vi "NT to Globals & XML.vi"(8 "Array":path[](array[path])) -> ()   [LabVIEW 2020]
uses:
  NT to XML Number.vi
  Globals/Dashboard_Cal_Globals.vi
  2021-MARS-Swerve/Globals/Intake_Globals.vi
panel:
  in  "NT Name Categories":string[](array[string])=["Turret", "Intake", "Magazine", "Flywheel", "FR", "FL", "BL", "BR", "Manual", "Cowl"]
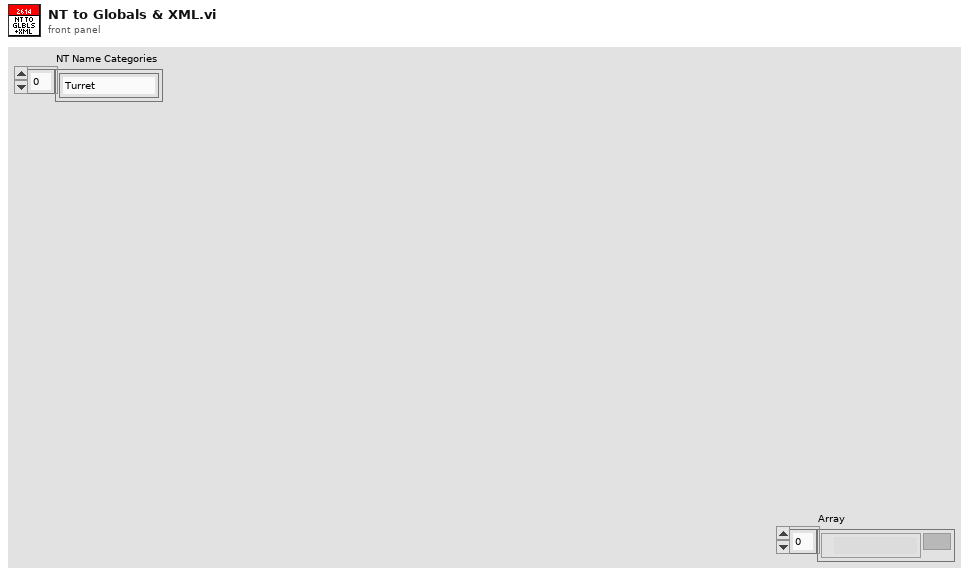
[diagram p1: front panel]
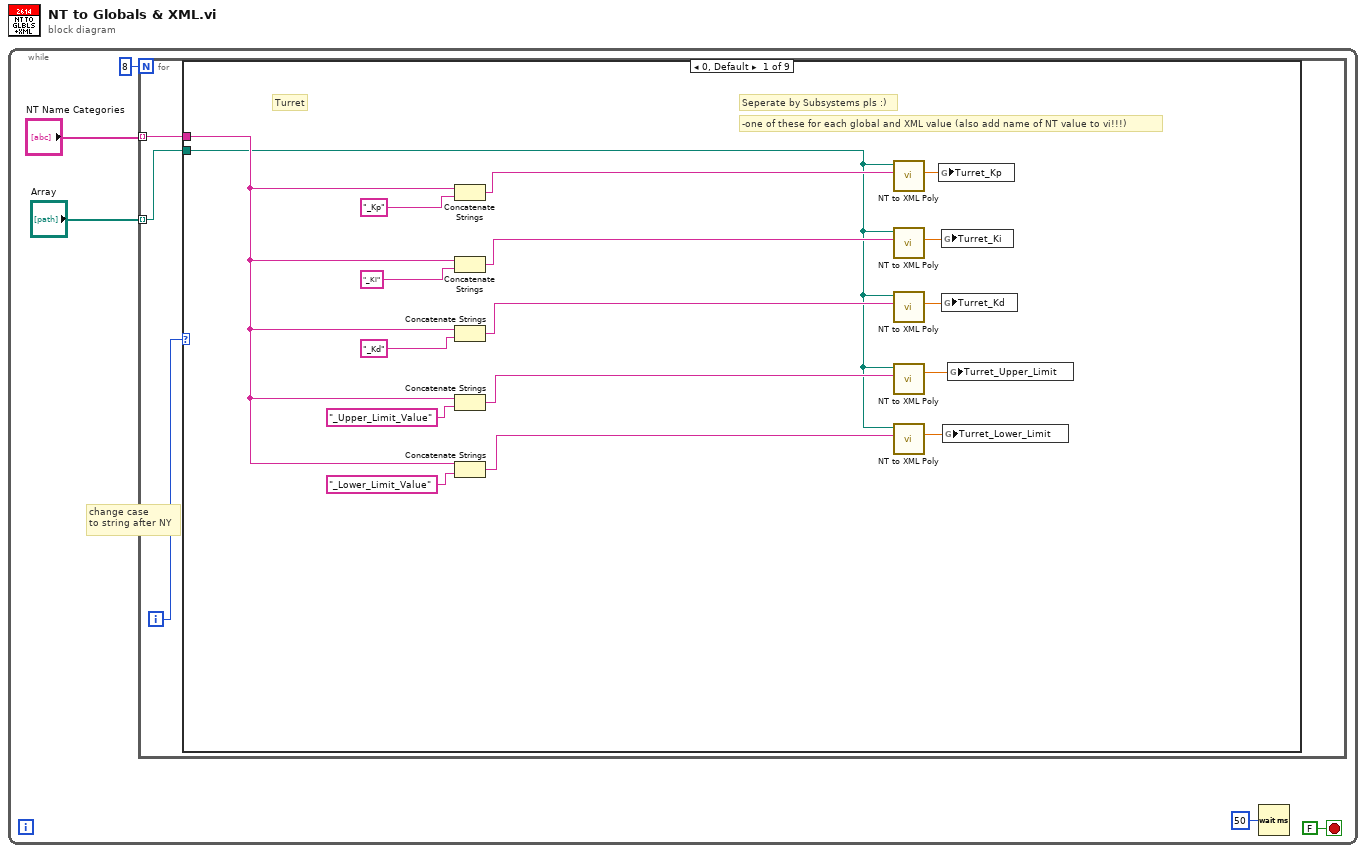
[diagram p0: block diagram]
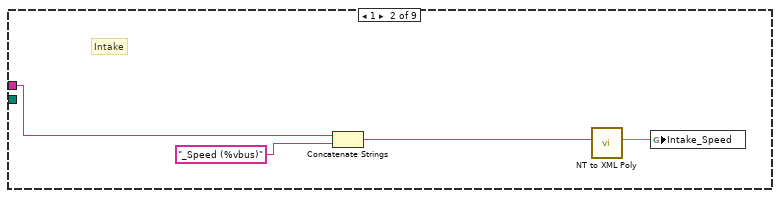
[diagram p2: hidden frame]
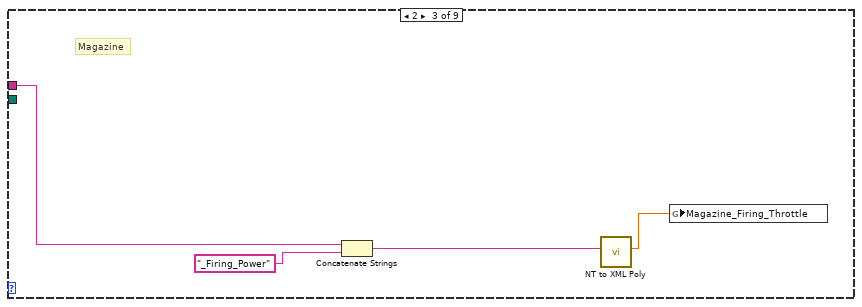
[diagram p3: hidden frame]
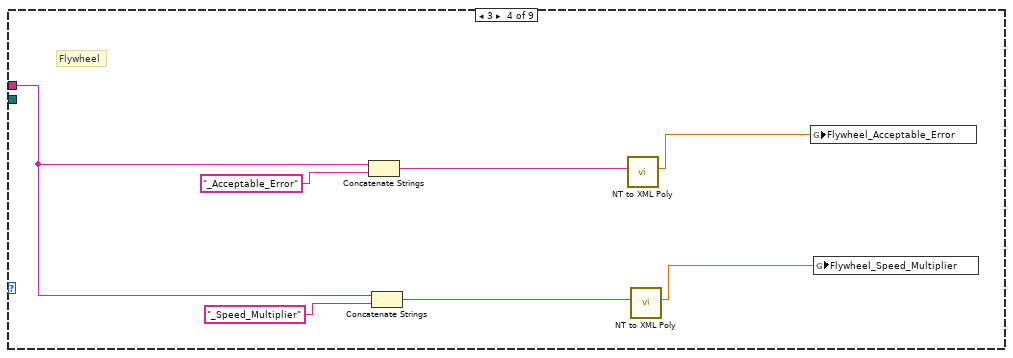
[diagram p4: hidden frame]
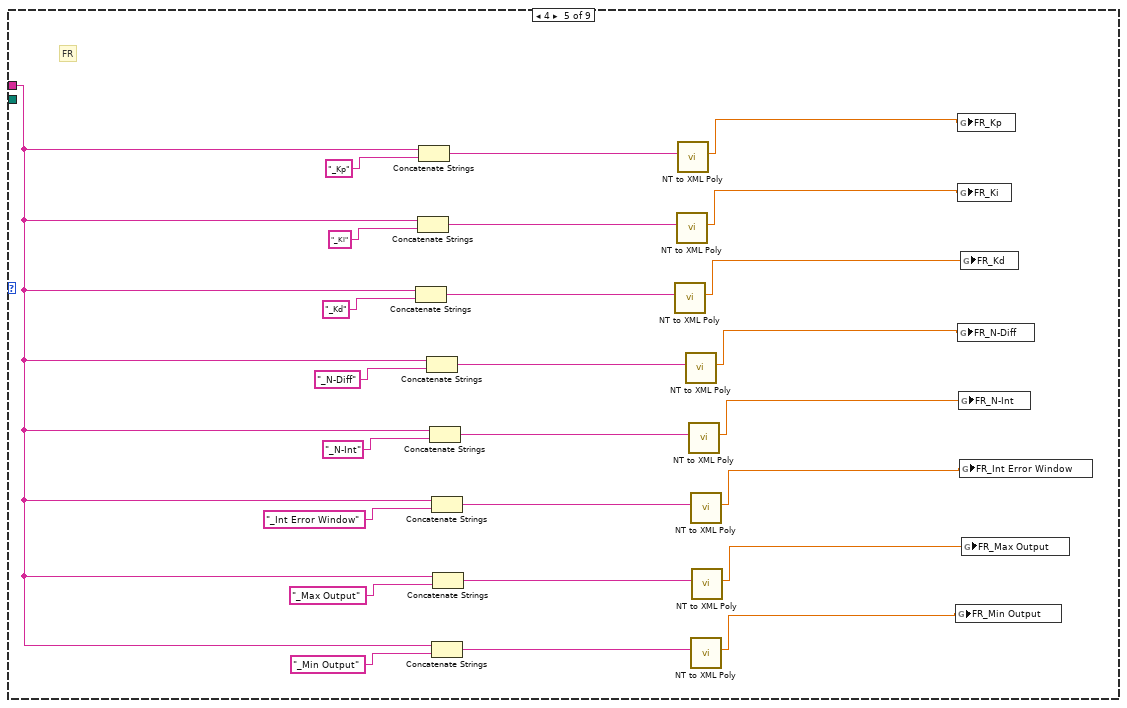
[diagram p5: hidden frame]
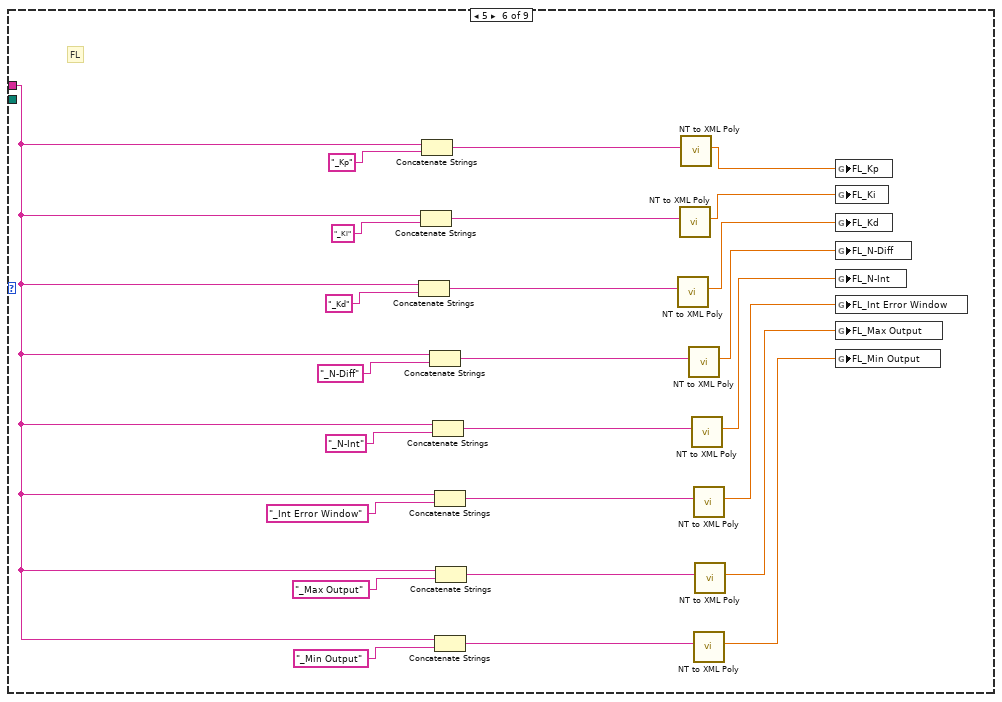
[diagram p6: hidden frame]
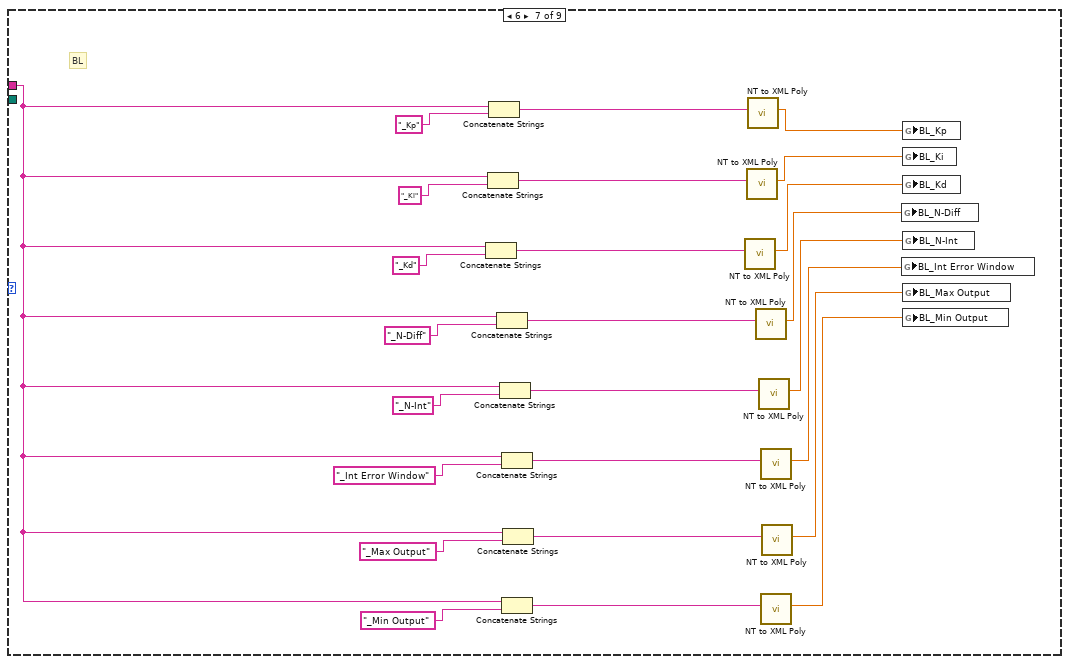
[diagram p7: hidden frame]
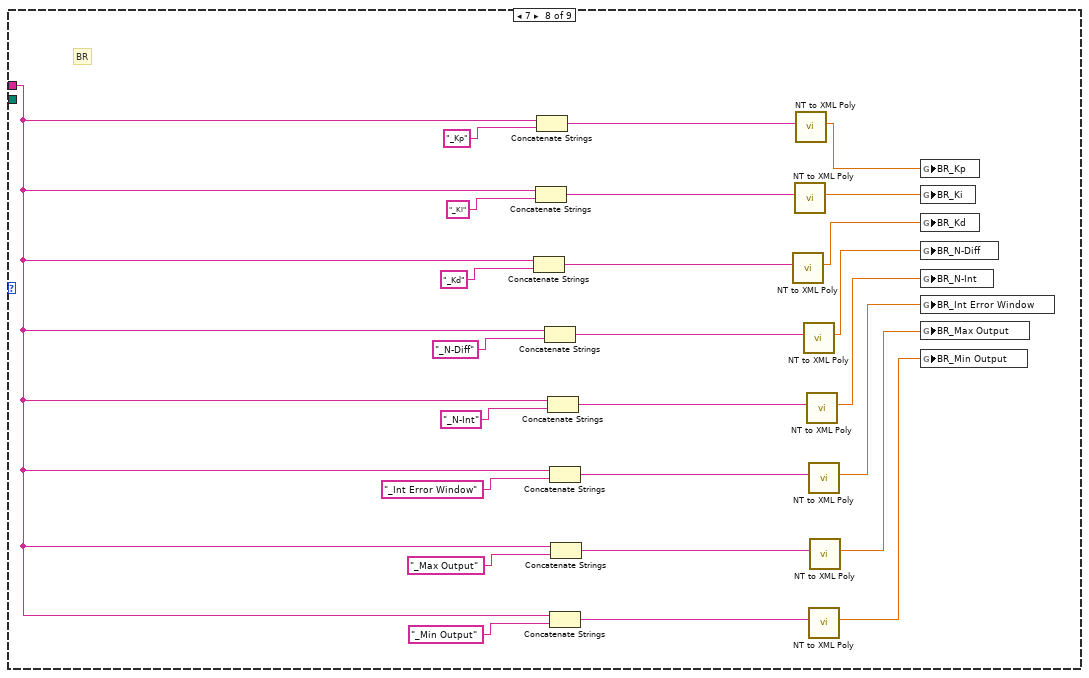
[diagram p8: hidden frame]
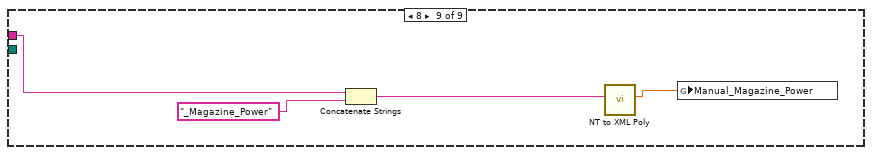
[diagram p9: hidden frame]
diagram:
  n1 = while {
    stop <- FALSE stop-if-true
    # "change case\nto string after NY"
    n2 = for {
      N: 8 -> [_]
      tunnel: "NT Name Categories" -> [w8] mode=indexing
      tunnel: "Array" -> [w7] mode=indexing
      i -> [w6]
      n3 = case shown="0, Default" w6 {
        tunnel: w8 -> [w15 w27 w31 w34 w41 w74 w99 w124 w141]
        tunnel: w7 -> [w9 _ _ _ _ _ _ _ _]
        frame 0, Default {
          # "Turret"
          # "-one of these for each global and XML value (also add name of NT value to vi!!!)"
          # "Seperate by Subsystems pls :)"
          n4 = Concatenate Strings(w15, "_Kp" ("NT Name")) -> (w14:string)
          n5 = Concatenate Strings(w15, "_Ki" ("NT Name")) -> (w13:string)
          n6 = Concatenate Strings(w15, "_Kd" ("NT Name")) -> (w12:string)
          n7 = Concatenate Strings(w15, "_Upper_Limit_Value" ("NT Name")) -> (w11:string)
          n8 = Concatenate Strings(w15, "_Lower_Limit_Value" ("NT Name")) -> (w10:string)
          n9 = call-poly "NT to XML Poly.vi"("NT Name"=w14, "XML File Path"=w9) -> ("Numeric"=w20:dbl)  [unwired: 9 in]
          n10 = call-poly "NT to XML Poly.vi"("NT Name"=w13, "XML File Path"=w9) -> ("Numeric"=w21:dbl)  [unwired: 9 in]
          n11 = call-poly "NT to XML Poly.vi"("NT Name"=w12, "XML File Path"=w9) -> ("Numeric"=w22:dbl)  [unwired: 9 in]
          n12 = call-poly "NT to XML Poly.vi"("NT Name"=w11, "XML File Path"=w9) -> ("Numeric"=w24:dbl)  [unwired: 9 in]
          n13 = call-poly "NT to XML Poly.vi"("NT Name"=w10, "XML File Path"=w9) -> ("Numeric"=w23:dbl)  [unwired: 9 in]
          n14 = global write "Dashboard_Cal_Globals.vi" "Turret_Kp"(w20) -> ()
          n15 = global write "Dashboard_Cal_Globals.vi" "Turret_Ki"(w21) -> ()
          n16 = global write "Dashboard_Cal_Globals.vi" "Turret_Kd"(w22) -> ()
          n17 = global write "Dashboard_Cal_Globals.vi" "Turret_Lower_Limit"(w23) -> ()
          n18 = global write "Dashboard_Cal_Globals.vi" "Turret_Upper_Limit"(w24) -> ()
        }
        frame 1 {
          # "Intake"
          n19 = Concatenate Strings(w27, "_Speed (%vbus)" ("NT Name")) -> (w28:string)
          n20 = call-poly "NT to XML Poly.vi"("NT Name"=w28) -> ("Numeric"=w26:dbl)  [unwired: 10 in]
          n21 = global write "Intake_Globals.vi" "Intake_Speed"(w26) -> ()
        }
        frame 2 {
          # "Magazine"
          n22 = Concatenate Strings(w31, "_Firing_Power" ("NT Name")) -> (w33:string)
          n23 = call-poly "NT to XML Poly.vi"("NT Name"=w33) -> ("Numeric"=w30:dbl)  [unwired: 10 in]
          n24 = global write "Dashboard_Cal_Globals.vi" "Magazine_Firing_Throttle"(w30) -> ()
        }
        frame 3 {
          # "Flywheel"
          n25 = Concatenate Strings(w34, "_Acceptable_Error" ("NT Name")) -> (w40:string)
          n26 = Concatenate Strings(w34, "_Speed_Multiplier" ("NT Name")) -> (w37:string)
          n27 = call-poly "NT to XML Poly.vi"("NT Name"=w40) -> ("Numeric"=w38:dbl)  [unwired: 10 in]
          n28 = call-poly "NT to XML Poly.vi"("NT Name"=w37) -> ("Numeric"=w35:dbl)  [unwired: 10 in]
          n29 = global write "Dashboard_Cal_Globals.vi" "Flywheel_Acceptable_Error"(w38) -> ()
          n30 = global write "Dashboard_Cal_Globals.vi" "Flywheel_Speed_Multiplier"(w35) -> ()
        }
        frame 4 {
          # "FR"
          n31 = Concatenate Strings(w41, "_Kd" ("NT Name")) -> (w61:string)
          n32 = Concatenate Strings(w41, "_Ki" ("NT Name")) -> (w63:string)
          n33 = Concatenate Strings(w41, "_Kp" ("NT Name")) -> (w65:string)
          n34 = Concatenate Strings(w41, "_N-Diff" ("NT Name")) -> (w59:string)
          n35 = Concatenate Strings(w41, "_N-Int" ("NT Name")) -> (w57:string)
          n36 = Concatenate Strings(w41, "_Int Error Window" ("NT Name")) -> (w55:string)
          n37 = Concatenate Strings(w41, "_Min Output" ("NT Name")) -> (w51:string)
          n38 = Concatenate Strings(w41, "_Max Output" ("NT Name")) -> (w53:string)
          n39 = call-poly "NT to XML Poly.vi"("NT Name"=w61) -> ("Numeric"=w47:dbl)  [unwired: 10 in]
          n40 = call-poly "NT to XML Poly.vi"("NT Name"=w63) -> ("Numeric"=w48:dbl)  [unwired: 10 in]
          n41 = call-poly "NT to XML Poly.vi"("NT Name"=w65) -> ("Numeric"=w49:dbl)  [unwired: 10 in]
          n42 = call-poly "NT to XML Poly.vi"("NT Name"=w59) -> ("Numeric"=w46:dbl)  [unwired: 10 in]
          n43 = call-poly "NT to XML Poly.vi"("NT Name"=w57) -> ("Numeric"=w45:dbl)  [unwired: 10 in]
          n44 = call-poly "NT to XML Poly.vi"("NT Name"=w55) -> ("Numeric"=w44:dbl)  [unwired: 10 in]
          n45 = call-poly "NT to XML Poly.vi"("NT Name"=w51) -> ("Numeric"=w42:dbl)  [unwired: 10 in]
          n46 = call-poly "NT to XML Poly.vi"("NT Name"=w53) -> ("Numeric"=w43:dbl)  [unwired: 10 in]
          n47 = global write "Dashboard_Cal_Globals.vi" "FR_Min Output"(w42) -> ()
          n48 = global write "Dashboard_Cal_Globals.vi" "FR_Kp"(w49) -> ()
          n49 = global write "Dashboard_Cal_Globals.vi" "FR_Ki"(w48) -> ()
          n50 = global write "Dashboard_Cal_Globals.vi" "FR_N-Diff"(w46) -> ()
          n51 = global write "Dashboard_Cal_Globals.vi" "FR_N-Int"(w45) -> ()
          n52 = global write "Dashboard_Cal_Globals.vi" "FR_Int Error Window"(w44) -> ()
          n53 = global write "Dashboard_Cal_Globals.vi" "FR_Kd"(w47) -> ()
          n54 = global write "Dashboard_Cal_Globals.vi" "FR_Max Output"(w43) -> ()
        }
        frame 5 {
          # "FL"
          n55 = Concatenate Strings(w74, "_Kd" ("NT Name")) -> (w86:string)
          n56 = Concatenate Strings(w74, "_Ki" ("NT Name")) -> (w88:string)
          n57 = Concatenate Strings(w74, "_Kp" ("NT Name")) -> (w90:string)
          n58 = Concatenate Strings(w74, "_N-Diff" ("NT Name")) -> (w84:string)
          n59 = Concatenate Strings(w74, "_N-Int" ("NT Name")) -> (w82:string)
          n60 = Concatenate Strings(w74, "_Int Error Window" ("NT Name")) -> (w80:string)
          n61 = Concatenate Strings(w74, "_Min Output" ("NT Name")) -> (w76:string)
          n62 = Concatenate Strings(w74, "_Max Output" ("NT Name")) -> (w78:string)
          n63 = call-poly "NT to XML Poly.vi"("NT Name"=w86) -> ("Numeric"=w71:dbl)  [unwired: 10 in]
          n64 = call-poly "NT to XML Poly.vi"("NT Name"=w88) -> ("Numeric"=w72:dbl)  [unwired: 10 in]
          n65 = call-poly "NT to XML Poly.vi"("NT Name"=w90) -> ("Numeric"=w73:dbl)  [unwired: 10 in]
          n66 = call-poly "NT to XML Poly.vi"("NT Name"=w84) -> ("Numeric"=w70:dbl)  [unwired: 10 in]
          n67 = call-poly "NT to XML Poly.vi"("NT Name"=w82) -> ("Numeric"=w69:dbl)  [unwired: 10 in]
          n68 = call-poly "NT to XML Poly.vi"("NT Name"=w80) -> ("Numeric"=w68:dbl)  [unwired: 10 in]
          n69 = call-poly "NT to XML Poly.vi"("NT Name"=w76) -> ("Numeric"=w66:dbl)  [unwired: 10 in]
          n70 = call-poly "NT to XML Poly.vi"("NT Name"=w78) -> ("Numeric"=w67:dbl)  [unwired: 10 in]
          n71 = global write "Dashboard_Cal_Globals.vi" "FL_Kp"(w73) -> ()
          n72 = global write "Dashboard_Cal_Globals.vi" "FL_Ki"(w72) -> ()
          n73 = global write "Dashboard_Cal_Globals.vi" "FL_Kd"(w71) -> ()
          n74 = global write "Dashboard_Cal_Globals.vi" "FL_N-Diff"(w70) -> ()
          n75 = global write "Dashboard_Cal_Globals.vi" "FL_N-Int"(w69) -> ()
          n76 = global write "Dashboard_Cal_Globals.vi" "FL_Int Error Window"(w68) -> ()
          n77 = global write "Dashboard_Cal_Globals.vi" "FL_Max Output"(w67) -> ()
          n78 = global write "Dashboard_Cal_Globals.vi" "FL_Min Output"(w66) -> ()
        }
        frame 6 {
          # "BL"
          n79 = Concatenate Strings(w99, "_Kd" ("NT Name")) -> (w111:string)
          n80 = Concatenate Strings(w99, "_Ki" ("NT Name")) -> (w113:string)
          n81 = Concatenate Strings(w99, "_Kp" ("NT Name")) -> (w115:string)
          n82 = Concatenate Strings(w99, "_N-Diff" ("NT Name")) -> (w109:string)
          n83 = Concatenate Strings(w99, "_N-Int" ("NT Name")) -> (w107:string)
          n84 = Concatenate Strings(w99, "_Int Error Window" ("NT Name")) -> (w105:string)
          n85 = Concatenate Strings(w99, "_Min Output" ("NT Name")) -> (w101:string)
          n86 = Concatenate Strings(w99, "_Max Output" ("NT Name")) -> (w103:string)
          n87 = call-poly "NT to XML Poly.vi"("NT Name"=w111) -> ("Numeric"=w96:dbl)  [unwired: 10 in]
          n88 = call-poly "NT to XML Poly.vi"("NT Name"=w113) -> ("Numeric"=w97:dbl)  [unwired: 10 in]
          n89 = call-poly "NT to XML Poly.vi"("NT Name"=w115) -> ("Numeric"=w98:dbl)  [unwired: 10 in]
          n90 = call-poly "NT to XML Poly.vi"("NT Name"=w109) -> ("Numeric"=w95:dbl)  [unwired: 10 in]
          n91 = call-poly "NT to XML Poly.vi"("NT Name"=w107) -> ("Numeric"=w94:dbl)  [unwired: 10 in]
          n92 = call-poly "NT to XML Poly.vi"("NT Name"=w105) -> ("Numeric"=w93:dbl)  [unwired: 10 in]
          n93 = call-poly "NT to XML Poly.vi"("NT Name"=w101) -> ("Numeric"=w91:dbl)  [unwired: 10 in]
          n94 = call-poly "NT to XML Poly.vi"("NT Name"=w103) -> ("Numeric"=w92:dbl)  [unwired: 10 in]
          n95 = global write "Dashboard_Cal_Globals.vi" "BL_N-Diff"(w95) -> ()
          n96 = global write "Dashboard_Cal_Globals.vi" "BL_Int Error Window"(w93) -> ()
          n97 = global write "Dashboard_Cal_Globals.vi" "BL_Kp"(w98) -> ()
          n98 = global write "Dashboard_Cal_Globals.vi" "BL_Ki"(w97) -> ()
          n99 = global write "Dashboard_Cal_Globals.vi" "BL_Kd"(w96) -> ()
          n100 = global write "Dashboard_Cal_Globals.vi" "BL_N-Int"(w94) -> ()
          n101 = global write "Dashboard_Cal_Globals.vi" "BL_Max Output"(w92) -> ()
          n102 = global write "Dashboard_Cal_Globals.vi" "BL_Min Output"(w91) -> ()
        }
        frame 7 {
          # "BR"
          n103 = Concatenate Strings(w124, "_Kd" ("NT Name")) -> (w135:string)
          n104 = Concatenate Strings(w124, "_Ki" ("NT Name")) -> (w134:string)
          n105 = Concatenate Strings(w124, "_Kp" ("NT Name")) -> (w133:string)
          n106 = Concatenate Strings(w124, "_N-Diff" ("NT Name")) -> (w136:string)
          n107 = Concatenate Strings(w124, "_N-Int" ("NT Name")) -> (w137:string)
          n108 = Concatenate Strings(w124, "_Int Error Window" ("NT Name")) -> (w138:string)
          n109 = Concatenate Strings(w124, "_Min Output" ("NT Name")) -> (w140:string)
          n110 = Concatenate Strings(w124, "_Max Output" ("NT Name")) -> (w139:string)
          n111 = call-poly "NT to XML Poly.vi"("NT Name"=w135) -> ("Numeric"=w121:dbl)  [unwired: 10 in]
          n112 = call-poly "NT to XML Poly.vi"("NT Name"=w134) -> ("Numeric"=w122:dbl)  [unwired: 10 in]
          n113 = call-poly "NT to XML Poly.vi"("NT Name"=w133) -> ("Numeric"=w123:dbl)  [unwired: 10 in]
          n114 = call-poly "NT to XML Poly.vi"("NT Name"=w136) -> ("Numeric"=w120:dbl)  [unwired: 10 in]
          n115 = call-poly "NT to XML Poly.vi"("NT Name"=w137) -> ("Numeric"=w119:dbl)  [unwired: 10 in]
          n116 = call-poly "NT to XML Poly.vi"("NT Name"=w138) -> ("Numeric"=w118:dbl)  [unwired: 10 in]
          n117 = call-poly "NT to XML Poly.vi"("NT Name"=w140) -> ("Numeric"=w116:dbl)  [unwired: 10 in]
          n118 = call-poly "NT to XML Poly.vi"("NT Name"=w139) -> ("Numeric"=w117:dbl)  [unwired: 10 in]
          n119 = global write "Dashboard_Cal_Globals.vi" "BR_Kp"(w123) -> ()
          n120 = global write "Dashboard_Cal_Globals.vi" "BR_Ki"(w122) -> ()
          n121 = global write "Dashboard_Cal_Globals.vi" "BR_Kd"(w121) -> ()
          n122 = global write "Dashboard_Cal_Globals.vi" "BR_N-Diff"(w120) -> ()
          n123 = global write "Dashboard_Cal_Globals.vi" "BR_N-Int"(w119) -> ()
          n124 = global write "Dashboard_Cal_Globals.vi" "BR_Int Error Window"(w118) -> ()
          n125 = global write "Dashboard_Cal_Globals.vi" "BR_Max Output"(w117) -> ()
          n126 = global write "Dashboard_Cal_Globals.vi" "BR_Min Output"(w116) -> ()
        }
        frame 8 {
          n127 = Concatenate Strings(w141, "_Magazine_Power" ("NT Name")) -> (w143:string)
          n128 = call-poly "NT to XML Poly.vi"("NT Name"=w143) -> ("Numeric"=w144:dbl)  [unwired: 10 in]
          n129 = global write "Dashboard_Cal_Globals.vi" "Manual_Magazine_Power"(w144) -> ()
        }
      }
    }
    n130 = Wait (ms)(milliseconds to wait=u32 50) -> ()  [unwired: 1 out]
  }
